vi "GT Clr Sts.vi"(8 "error in (no error)":errorcluster caption="错误输入（无错误）", 9 "count":i16, 10 "axis":i16, 11 "cardNum":i16) -> (0 "error out":errorcluster caption="错误输出", 3 "function return":i16)   [LabVIEW 2014, in "gts.lvlib"]
doc: "GT_API GT_ClrSts(short cardNum,short axis,short count=1);"
uses:
  gts.lvlib
  gts.dll
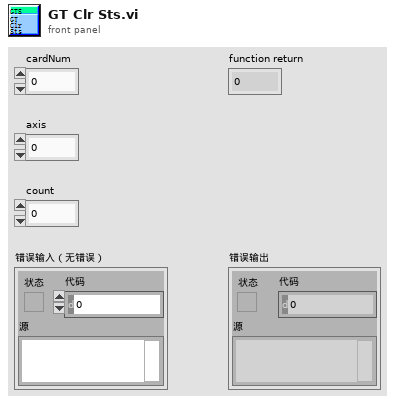
[diagram p1: front panel]
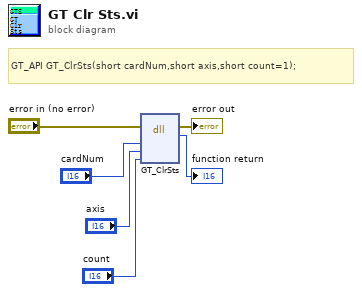
[diagram p0: block diagram]
diagram:
  # "GT_API GT_ClrSts(short cardNum,short axis,short count=1);"
  n1 = dll-call lib="PTH2>abs F.多卡库-控制卡基本运动例程(labview)gts.*" fn="GT_ClrSts"(error in="error in (no error)", "cardNum"="cardNum", "axis"="axis", "count"="count") -> (error out=→"error out":errorcluster, →"function return":i16)  [unwired: 5 in, 1 out]
